vi "Inline Rx Start.vi"(8 "error in (no error)":errorcluster, 10 "Dispatcher Interface in":refnum<class "Dispatcher Interface.lvclass">, 11 "Plugin Timing Group in":refnum<class "Plugin Timing.lvclass">) -> (0 "error out":errorcluster, 2 "Dispatcher Interface out":refnum<class "Dispatcher Interface.lvclass">, 3 "Plugin Timing Group out":refnum<class "Plugin Timing.lvclass">)   [LabVIEW 2017, in "DSF Core.lvlib" / "Plugin Timing.lvclass"]
uses:
  Plugin Timing.lvclass
  Interfaces/Dispatcher/Dispatcher Interface.lvclass
  Plugin Timing.lvclass/Plugin Timing.ctl
  Timing.lvclass/Timing.ctl
  Transfer Group Timing.lvclass/Transfer Group Timing.ctl
  Transfer Group Timing.lvclass
  C:/Git/DSF/Data Sharing Framework/Source/Core/Engine/Classes/Timing/Timing.lvclass
  Timing.lvclass
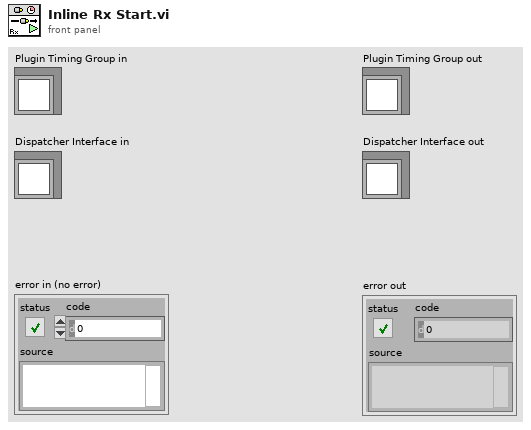
[diagram p1: front panel]
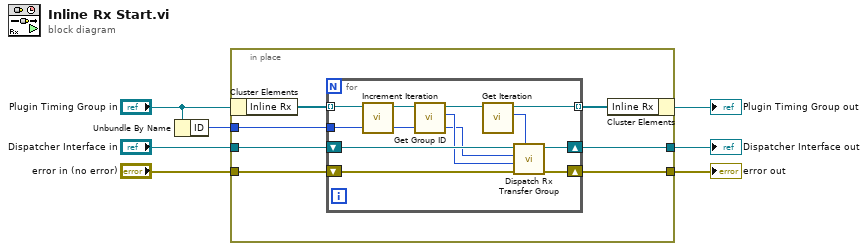
[diagram p0: block diagram]
diagram:
  n1 = Unbundle By Name("Plugin Timing Group in") -> ("ID"=w1:i32)
  n2 = in-place {
    in-place-border: "Dispatcher Interface in" -> [w12]
    in-place-border: [w11] -> w5
    in-place-border: [w10] -> w3
    in-place-border: "error in (no error)" -> [w9]
    in-place-border: w1 -> [w8]
    n3 = in-place-cluster #1("Plugin Timing Group in") -> ("Inline Rx"=w14:refnum<class "Transfer Group Timing.lvclass">[])
    n4 = for {
      tunnel: w14 -> [w18] mode=indexing
      tunnel: [w22] -> w13 mode=indexing
      shift-right: [w25] -> w11
      shift-left: w12 -> [w19]
      shift-right: [w24] -> w10
      shift-left: w9 -> [w20]
      tunnel: w8 -> [w15]
      n5 = call "Increment Iteration.vi"("Timing in"=w18) -> ("Timing out"=w17:refnum<class "Transfer Group Timing.lvclass">)  [unwired: 10 in]
      n6 = call "Get Group ID.vi"("Transfer Group Timing in"=w17) -> ("Group ID"=w16:i32, "Transfer Group Timing out"=w23:refnum<class "Transfer Group Timing.lvclass">)  [unwired: 9 in]
      n7 = call "Get Iteration.vi"("Timing in"=w23) -> ("Iteration"=w21:u64, "Timing out"=w22:refnum<class "Transfer Group Timing.lvclass">)  [unwired: 9 in]
      n8 = call "Dispatch Rx Transfer Group.vi"("Iteration"=w21, "error in (no error)"=w20, "Transfer Group ID"=w16, "Plugin ID"=w15, "Dispatcher Interface in"=w19) -> ("error out"=w24:errorcluster, "Dispatcher Interface out"=w25:refnum<class "Dispatcher Interface.lvclass">)  [unwired: 5 in]
    }
    n9 = in-place-cluster #1("Inline Rx"=w13) -> (→"Plugin Timing Group out":refnum<class "Plugin Timing.lvclass">)
  }
  "Dispatcher Interface out" <- w5
  "error out" <- w3
